vi "ROI entry-ROI shift dialogue.vi"() -> (3 "Cancelled (Left button pressed)":bool)   [LabVIEW 2017]
uses:
  Globals/gl_ROI Entry UI globals.vi
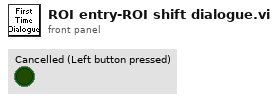
[diagram p1: front panel]
types:
  T1 = typedef "ROI entry screen ctrl refs cluster.ctl" = cluster{"Done button":refnum<vi>, "Imaging button":refnum<vi>, "Acquisition button":refnum<vi>, "POI dwell time (us)":refnum<vi>, "Scan dwell time per pixel (us)":refnum<vi>, "# of planes":refnum<vi>, "Zoom Ctrl":refnum<vi>, "Equal size":refnum<vi>, "Channel":refnum<vi>, "Image Display":refnum<vi>, "Z-Plane Selector":refnum<vi>, "Number of lines left":refnum<vi>, "Z-stack folder path":refnum<vi>, "POI Density":refnum<vi>, "Arb Plane Entry":refnum<vi>, "Whole plane":refnum<vi>, "Clear Last":refnum<vi>, "Clear All":refnum<vi>, "Trial Length (sec)":refnum<vi>, "Palette Type":refnum<vi>, "Intensity slider":refnum<vi>, "# POI":refnum<vi>, "Max Z Proj":refnum<vi>, "Zplane ind":refnum<vi>, "Wavelength (nm)":refnum<vi>, "Number of Trials":refnum<vi>, "Funct stim.trig.enable":refnum<vi>, "Funct stim.trig.delay (s)":refnum<vi>, "Line Mode":refnum<vi>, "Step size (µm)":refnum<vi>, "ROI move mode":refnum<vi>, "Cool-down time (s)":refnum<vi>, "Enable cool-down time":refnum<vi>, "Motor Z ind. (um)":refnum<vi>, "AOL Z ind. (um)":refnum<vi>, "Load Reference Image":refnum<vi>}
  T2 = typedef "ROI move mode.ctl" = enum16{"ROI on ALL planes", "ROI on current plane"}
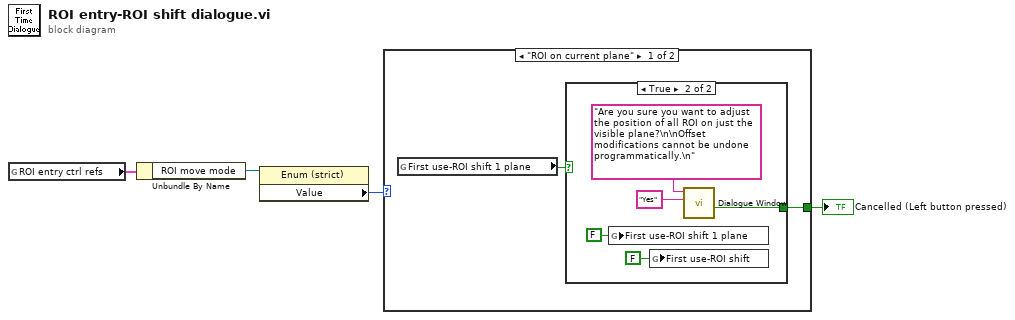
[diagram p0: block diagram]
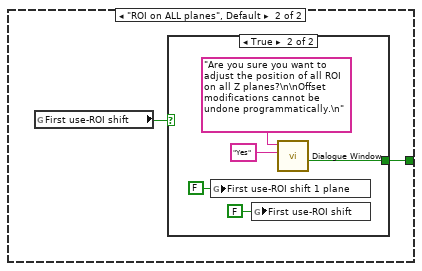
[diagram p3: hidden frame]
diagram:
  n1 = global read "gl_ROI Entry UI globals.vi" "ROI entry ctrl refs"() -> (w2:T1)
  n2 = Unbundle By Name(w2) -> ("ROI move mode"=w3:refnum<vi>)
  n3 = property class="Enum (strict)"(reference=w3) -> ("Value"=w4:T2)  [unwired: 1 in, 2 out]
  n4 = case shown="\"ROI on current plane\"" w4 {
    tunnel: [w5 w12] -> w1
    frame "ROI on current plane" {
      n5 = global read "gl_ROI Entry UI globals.vi" "First use-ROI shift 1 plane"() -> (w6:bool)
      n6 = case shown="True" w6 {
        tunnel: [_ w7] -> w5
        frame False {
        }
        frame True {
          n7 = global write "gl_ROI Entry UI globals.vi" "First use-ROI shift 1 plane"(FALSE ("First use-ROI shift")) -> ()
          n8 = global write "gl_ROI Entry UI globals.vi" "First use-ROI shift"(FALSE ("First use-ROI shift")) -> ()
          n9 = call "Dialogue Window.vi"("Caption-Right button (OK)"="Yes", "Message string"="Are you sure you want to adjust the position of all ROI on just the visible plane?\n\nOffset modifications cannot be undone programmatically.\n") -> ("Cancelled (Left button pressed)"=w7:bool)  [unwired: 7 in, 2 out]
        }
      }
    }
    frame "ROI on ALL planes", Default {
      n10 = global read "gl_ROI Entry UI globals.vi" "First use-ROI shift"() -> (w13:bool)
      n11 = case shown="True" w13 {
        tunnel: [_ w14] -> w12
        frame False {
        }
        frame True {
          n12 = global write "gl_ROI Entry UI globals.vi" "First use-ROI shift 1 plane"(FALSE ("First use-ROI shift")) -> ()
          n13 = global write "gl_ROI Entry UI globals.vi" "First use-ROI shift"(FALSE ("First use-ROI shift")) -> ()
          n14 = call "Dialogue Window.vi"("Caption-Right button (OK)"="Yes", "Message string"="Are you sure you want to adjust the position of all ROI on all Z planes?\n\nOffset modifications cannot be undone programmatically.\n") -> ("Cancelled (Left button pressed)"=w14:bool)  [unwired: 7 in, 2 out]
        }
      }
    }
  }
  "Cancelled (Left button pressed)" <- w1
